vi "Read Analogue.vi"(8 "error in (no error)":errorcluster, 11 "PS Instrument":refnum<class "Power Supply Instrument.lvclass">) -> (0 "error out":errorcluster, 2 "Waveforms":waveform(dbl)[](array[waveform]), 3 "PS Instrument out":refnum<class "Power Supply Instrument.lvclass">)   [LabVIEW 2025, in "Power Supply.lvlib" / "Power Supply Instrument.lvclass"]
uses:
  Power Supply Instrument.lvclass
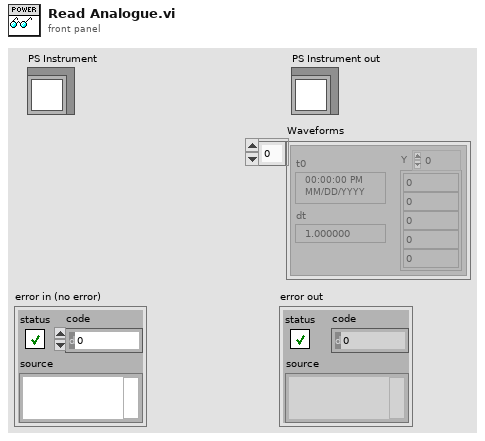
[diagram p1: front panel]
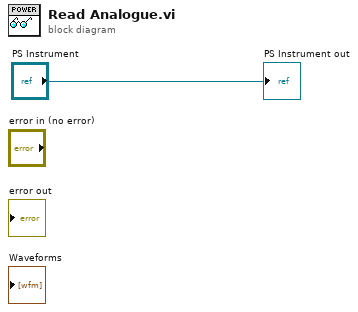
[diagram p0: block diagram]
diagram:
  "PS Instrument out" <- "PS Instrument"
